vi "waveCase.vi"() -> ()   [LabVIEW 2015]
uses:
  <vilib>/Analysis/NI_AALBase.lvlib
panel:
  in  "frequency":dbl(knob)=0.0078125 scale=0.0..10.0
  in  "amplitude":dbl(slide)=1.0 scale=0.0..10.0
  in  "Signal":string(combo)
  out "Waveform Chart":dbl[](graph)
  in  "Stop Button":bool
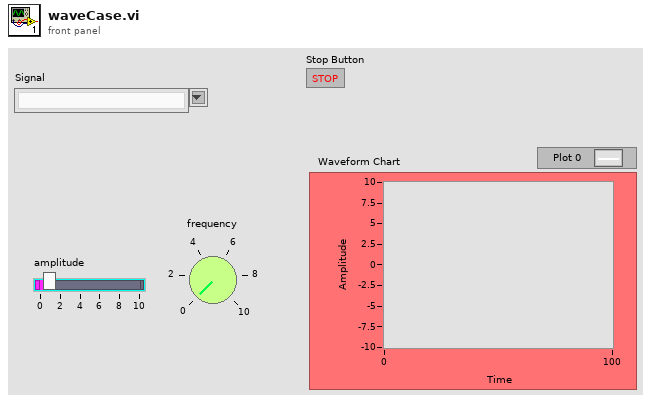
[diagram p1: front panel]
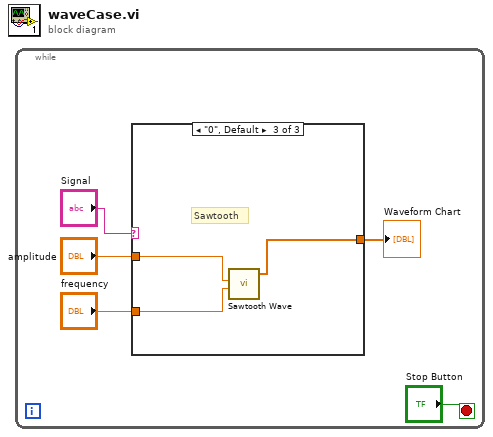
[diagram p0: block diagram]
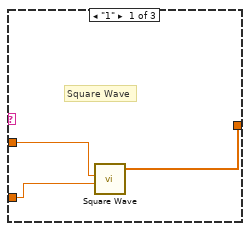
[diagram p2: hidden frame]
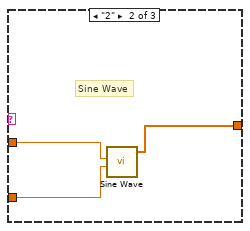
[diagram p3: hidden frame]
diagram:
  n1 = while {
    stop <- "Stop Button" stop-if-true
    n2 = case shown="\"0\", Default" "Signal" {
      tunnel: [w8 w11 w14] -> w3
      tunnel: "amplitude" -> [w6 w10 w13]
      tunnel: "frequency" -> [w7 w9 w12]
      frame "1" {
        # "Square Wave"
        n3 = call <vilib>:"Square Wave.vi"("amplitude"=w6, "frequency"=w7) -> ("square wave"=w8:dbl[])  [unwired: 4 in, 2 out]
      }
      frame "2" {
        # "Sine Wave"
        n4 = call <vilib>:"Sine Wave.vi"("amplitude"=w10, "frequency"=w9) -> ("sine wave"=w11:dbl[])  [unwired: 3 in, 2 out]
      }
      frame "0", Default {
        # "Sawtooth"
        n5 = call <vilib>:"Sawtooth Wave.vi"("amplitude"=w13, "frequency"=w12) -> ("sawtooth wave"=w14:dbl[])  [unwired: 3 in, 2 out]
      }
    }
    "Waveform Chart" <- w3
  }
